vi "Strip Comments.vi"(1 "?":string) -> (0 "?":string)   [LabVIEW 2020]
doc: "Author: Scott Hannahs <sth@magnet.fsu.edu>\nCopyright 2018 Florida State University, All rights reserved."
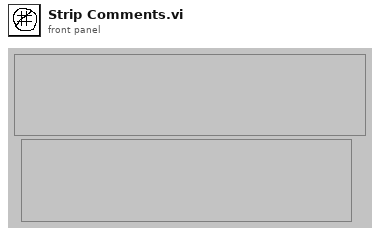
[diagram p1: front panel]
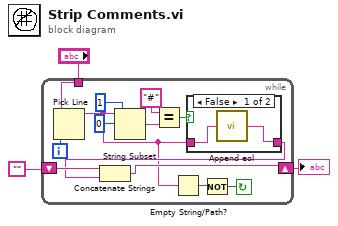
[diagram p0: block diagram]
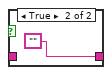
[diagram p2: hidden frame]
diagram:
  n1 = while {
    tunnel: "?" -> [w15]
    shift-left: "" -> [w14]
    shift-right: [w13] -> w1
    i -> [w16]
    stop <- w4 continue-if-true
    n2 = Pick Line(multi-line string=w15, line index=w16) -> (output string=w6:string)  [unwired: 1 in]
    n3 = String Subset(string=w6, offset (0)=0, length (rest)=1) -> (substring=w10:string)
    n4 = Equal?(x="#", y=w10) -> (x = y?=w8:bool)
    n5 = Empty String/Path?(string/path=w6) -> (empty?=w5:bool)
    n6 = case shown="False" w8 {
      tunnel: [w17 ""] -> w7
      tunnel: w6 -> [w18 _]
      frame False {
        n7 = call "Append eol.vi"("INPUT STRING"=w18) -> ("OUTPUT STRING (PLUS End of Line)"=w17:string)
      }
      frame True {
      }
    }
    n8 = Concatenate Strings(w14, w7) -> (w13:string)
    n9 = Not(x=w5) -> (.not. x?=w4:bool)
  }
  "?" <- w1
